vi "Write Log Data.vi"(8 "error in (no error)":errorcluster, 10 "Log Data":T1, 11 "CSV in":refnum<class "CSV.lvclass">) -> (0 "error out":errorcluster, 3 "CSV out":refnum<class "CSV.lvclass">)   [LabVIEW 2017, in "Report_lib.lvlib" / "CSV.lvclass"]
uses:
  CSV.lvclass
  CSV.lvclass/CSV.ctl
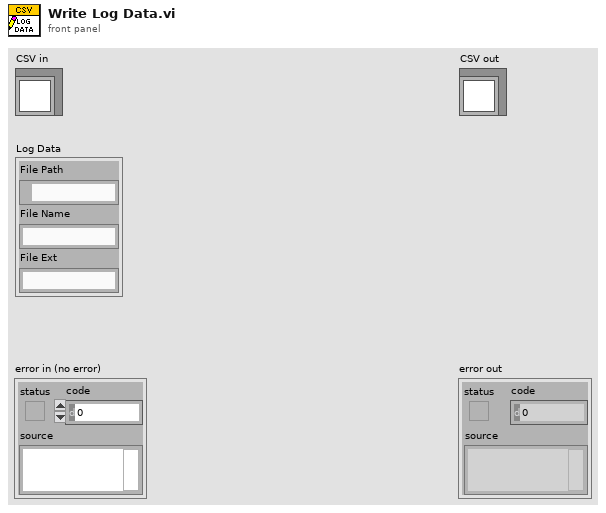
[diagram p1: front panel]
types:
  T1 = cluster{"File Path":path, "File Name":string, "File Ext":string}
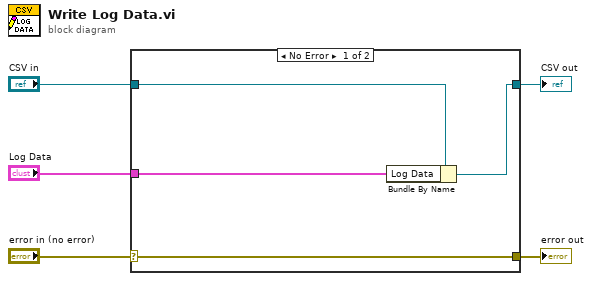
[diagram p0: block diagram]
diagram:
  n1 = case shown="No Error" "error in (no error)" {
    selector: "error in (no error)" -> [w9 w10]
    tunnel: [w9 w10] -> w4
    tunnel: [w7 w11] -> w2
    tunnel: "CSV in" -> [w8 w11]
    tunnel: "Log Data" -> [w6 _]
    frame No Error {
      n2 = Bundle By Name(cluster=w8, "Log Data"=w6) -> (w7:refnum<class "CSV.lvclass">)
    }
    frame Error {
    }
  }
  "error out" <- w4
  "CSV out" <- w2
